vi "Bang_Bang_LOX.vi"() -> ()   [LabVIEW 2019]
uses:
  <vilib>/Instr/_visa.llb/VISA Configure Serial Port (Instr).vi
panel:
  in  "Blank Button":bool
  in  "Pruseure":string
  in  "stop":bool
  out "Waveform Chart":dbl(graph)
  in  "COM PORT":string(combo)
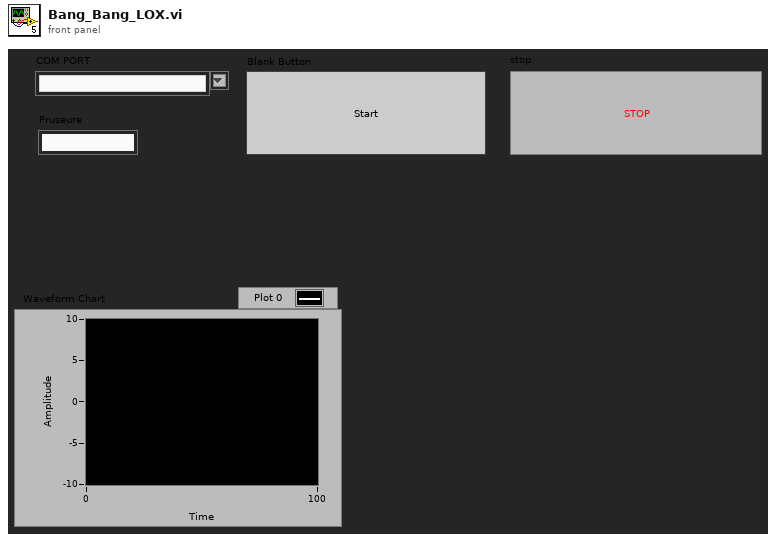
[diagram p1: front panel]
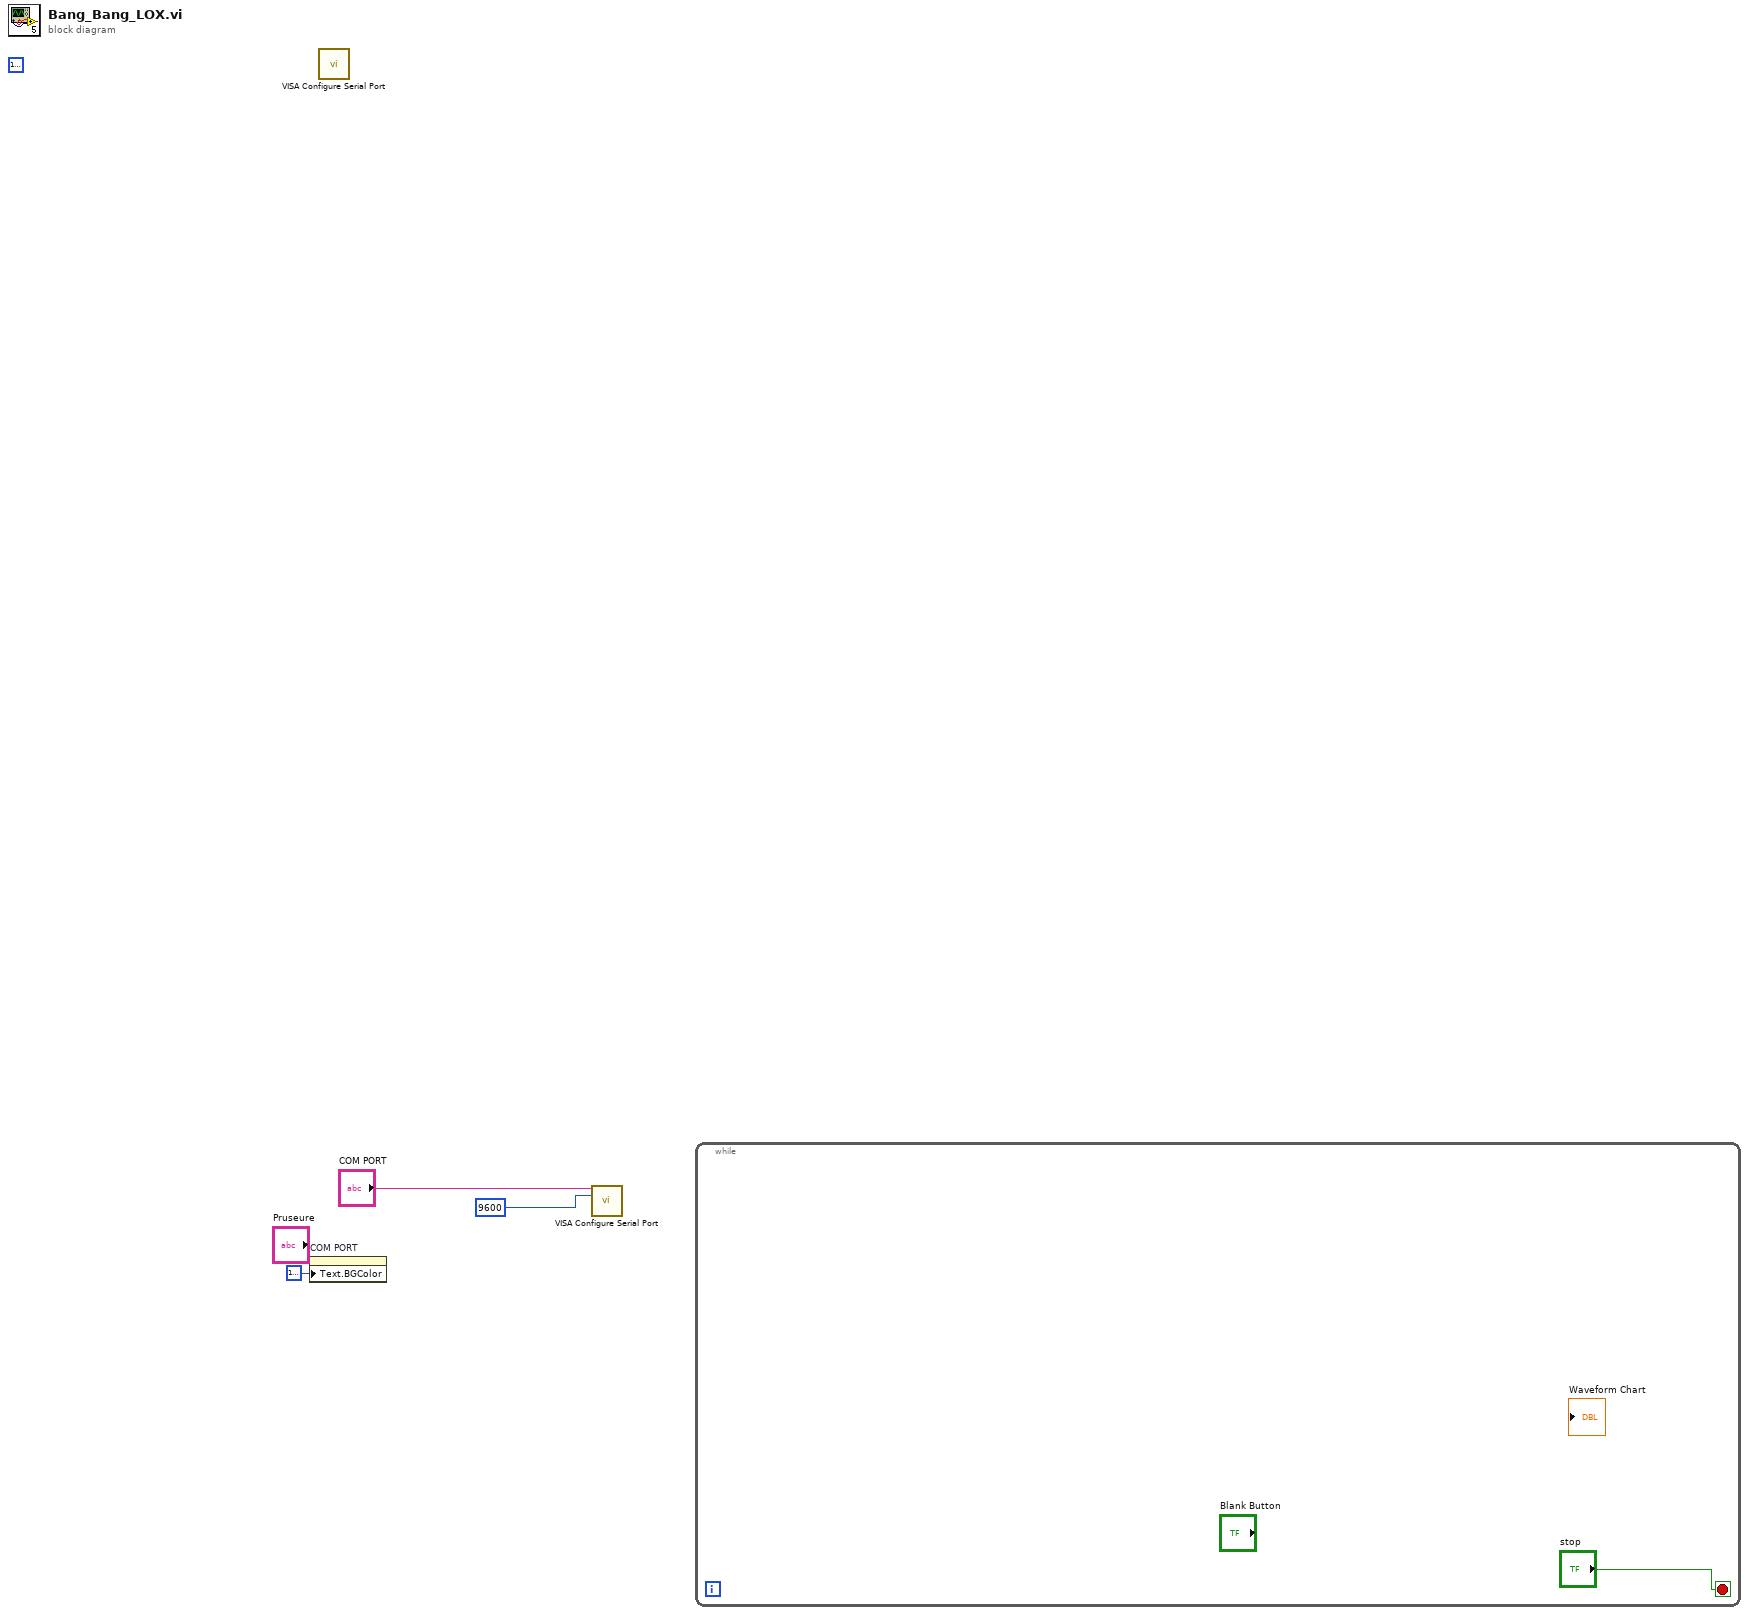
[diagram p0: block diagram]
diagram:
  w4 = u32 16777226 ("Text.Text Colors:BG Color")
  n1 = property on="COM PORT" class="CmbBox"("Text.BGColor"=u32 16777226 ("Text.Text Colors:BG Color")) -> ()  [unwired: 2 in, 2 out]
  n2 = call-poly "VISA Configure Serial Port"() -> ("VISA resource name"=w5:refnum<visa-resource-name>)  [unwired: 13 in, 2 out]
  n3 = call-poly "VISA Configure Serial Port"("VISA resource name"="COM PORT", "baud rate (9600)"=u32 9600) -> ()  [unwired: 12 in, 2 out]
  n4 = while {
    stop <- "stop" stop-if-true
  }
